vi "DIO Readback.vi"(7 "Box ID":u8, 8 "error in (no error)":errorcluster, 11 "ENET in":refnum<class "ENET_BS120x.lvclass">) -> (0 "error out":errorcluster, 2 "DIO Readback":bool[](array[boolean]), 3 "ENET out":refnum<class "ENET_BS120x.lvclass">)   [LabVIEW 2021, in "BS120x Driver.lvlib" / "ENET_BS120x.lvclass"]
uses:
  ENET_BS120x.lvclass
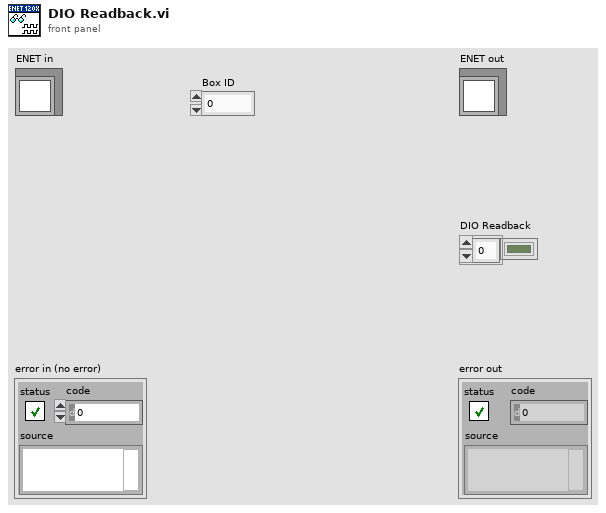
[diagram p1: front panel]
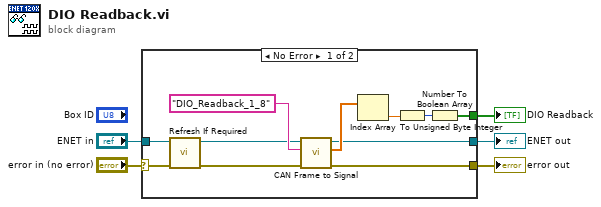
[diagram p0: block diagram]
diagram:
  n1 = case shown="No Error" "error in (no error)" {
    selector: "error in (no error)" -> [w9 w17]
    tunnel: [w16 w17] -> w5
    tunnel: [w11 w18] -> w4
    tunnel: [w10 _] -> w3
    tunnel: "ENET in" -> [w7 w18]
    frame No Error {
      n2 = call "Refresh If Required.vi"("error in (no error)"=w9, "Ethernet in"=w7) -> ("error out"=w8:errorcluster, "Ethernet out"=w6:refnum<class "ENET_BS120x.lvclass">)  [unwired: 8 in]
      n3 = call "CAN Frame to Signal.vi"("error in (no error)"=w8, "Frame"="DIO_Readback_1_8", "ENET in"=w6) -> ("error out"=w16:errorcluster, "signal data"=w12:dbl[], "ENET out"=w11:refnum<class "ENET_BS120x.lvclass">)  [unwired: 6 in]
      n4 = Index Array(array=w12) -> (element=w13:dbl)  [unwired: 1 in]
      n5 = To Unsigned Byte Integer(number=w13) -> (unsigned 8bit integer=w14:u8)
      n6 = Number To Boolean Array(number=w14) -> (Boolean array=w10:bool[])
    }
    frame Error {
    }
  }
  "error out" <- w5
  "ENET out" <- w4
  "DIO Readback" <- w3
